vi "WMPlayer.vi"() -> ()   [LabVIEW 2021]
panel:
  in  "Path":path
  in  "WindowsMediaPlayer":refnum<k7>(container)
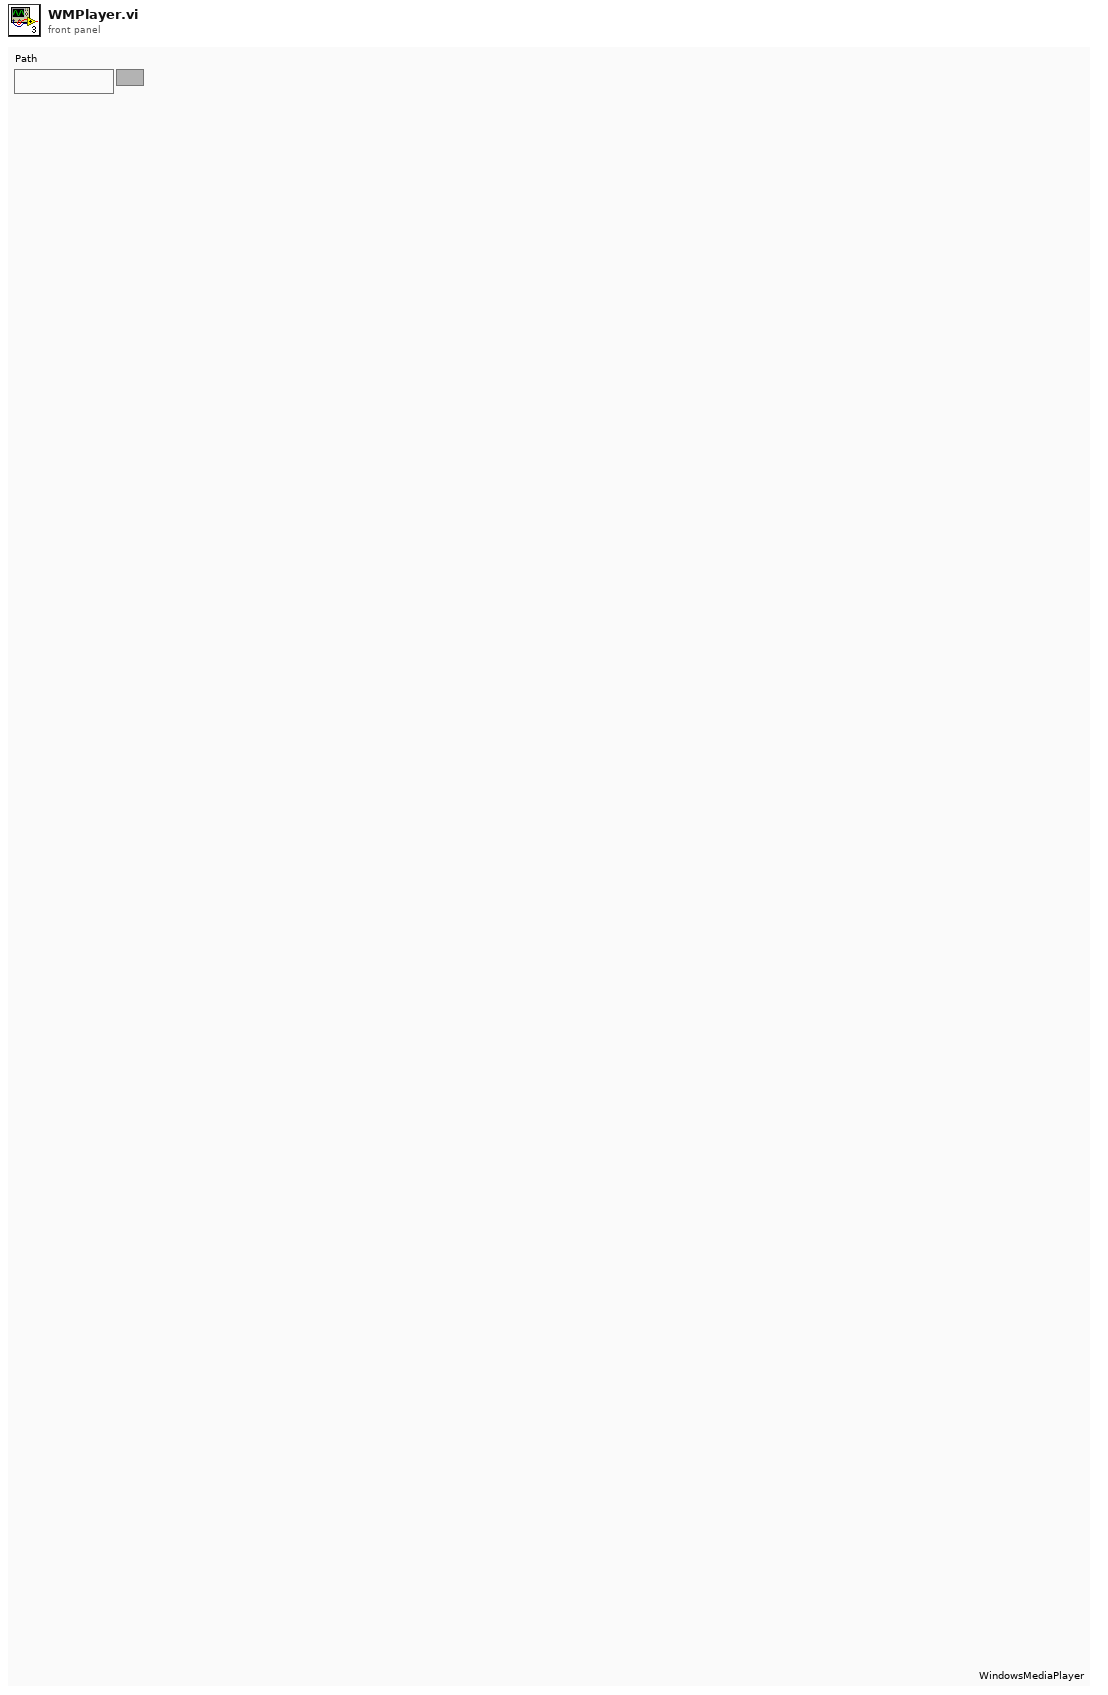
[diagram p1: front panel]
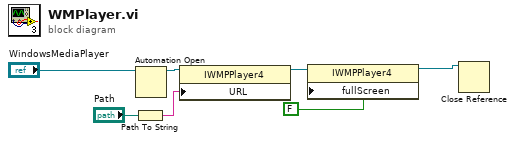
[diagram p0: block diagram]
diagram:
  n1 = Path To String(path="Path") -> (string=w5:string)
  n2 = Automation Open(Automation Refnum="WindowsMediaPlayer") -> (Automation Refnum=w6:refnum<k7>)  [unwired: 3 in, 1 out]
  n3 = property class="IWMPPlayer4"(reference=w6, "URL"=w5) -> (reference out=w3:refnum<k7>)  [unwired: 1 in, 1 out]
  n4 = property class="IWMPPlayer4"(reference=w3, "fullScreen"=FALSE) -> (reference out=w1:refnum<k7>)  [unwired: 1 in, 1 out]
  n5 = Close Reference(reference=w1) -> ()  [unwired: 1 in, 1 out]
